vi "Read Editor Position from INI.vi"(8 "error in":errorcluster) -> (0 "error out":errorcluster, 1 "Use Size":bool, 2 "Bounds Valid":bool, 3 "Window Bounds":T1)   [LabVIEW 2021, in "lv_icon.lvlib"]
doc: "Reads the position from the INI file and converts it to a window position cluster."
uses:
  <vilib>/LabVIEW Icon API/lv_icon/lv_icon.lvlib
  <vilib>/Utility/miscctls.llb/LVRectTypeDef.ctl
  <resource>/dialog/lvconfig.llb/LV Config Read Boolean.vi
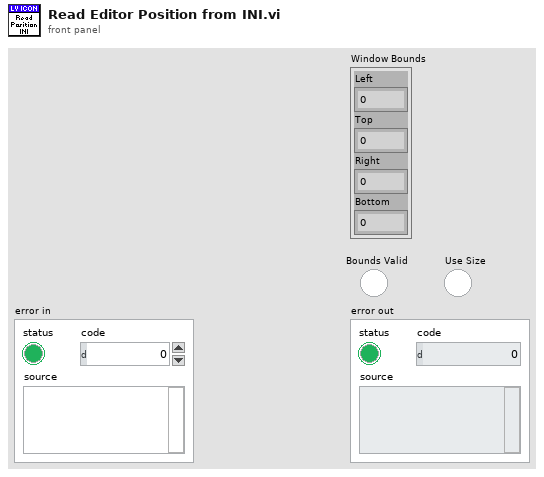
[diagram p1: front panel]
types:
  T1 = typedef "LVRectTypeDef.ctl" = cluster{"Left":i16, "Top":i16, "Right":i16, "Bottom":i16}
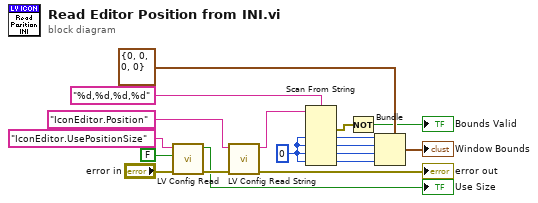
[diagram p0: block diagram]
diagram:
  w12 = i16 0 ("default value 1")
  n1 = call-poly <resource>:"LV Config Read.vi"("error in"="error in", "default value"=FALSE, "key"="IconEditor.UsePositionSize") -> ("error out"=w17:errorcluster, "value"=→"Use Size":bool)  [unwired: 2 in, 1 out]
  n2 = call <resource>:"LV Config Read String.vi"("error in"=w17, "key"="IconEditor.Position") -> ("error out"=→"error out":errorcluster, "value"=w14:string)  [unwired: 3 in, 1 out]
  n3 = Scan From String(format string="%d,%d,%d,%d", input string=w14, default 1=w12, default 2=w12, default 3=w12, default 4=w12) -> (error out=w18:errorcluster, output 1=w9:i16, output 2=w8:i16, output 3=w7:i16, output 4=w6:i16)  [unwired: 2 in, 2 out]
  n4 = Not(x=w18) -> (.not. x?=→"Bounds Valid":bool)
  n5 = Bundle(cluster=T1 {"Left"=0, "Top"=0, "Right"=0, "Bottom"=0} ("Front Panel Window:Window Bounds"), "Left"=w9, "Top"=w8, "Right"=w7, "Bottom"=w6) -> (→"Window Bounds":T1)
